vi "DropVI_SimpleClientPublisher.vi"() -> ()   [LabVIEW 2013, in "MQTT Client.lvlib"]
uses:
  MQTT Client.lvlib
  <vilib>/LabVIEW Open Source Project/MQTT Connection/MQTT_Connection/Connection/Connection.lvclass
  Client class/Client.lvclass/Client.ctl
  <vilib>/LabVIEW Open Source Project/MQTT Connection/MQTT_Base/Base Class/MQTT_Base.lvclass/MQTT_Base.ctl
  <vilib>/LabVIEW Open Source Project/MQTT Control Packets/Control Packets/PUBLISH/PUBLISH.lvclass
  Client class/Client.lvclass
  <vilib>/LabVIEW Open Source Project/MQTT Connection/MQTT_Base/Base Class/MQTT_Base.lvclass
panel:
  out "last error":errorcluster
  in  "Connection":bool
  out "Waveform Chart":dbl(graph)
  out "Published":bool
  in  "Stop Client":bool
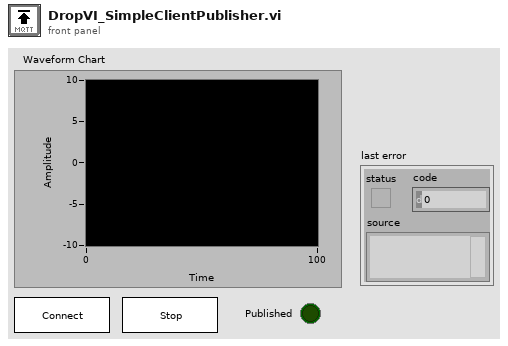
[diagram p1: front panel]
types:
  T1 = typedef "MQTT Client.lvlib/Client.lvclass/Public Events -- cluster.ctl" = cluster{"Connection Status":refnum<user-event>, "Connected":refnum<user-event>, "Application Message":refnum<user-event>}
  T2 = typedef "MQTT Base.lvlib/MQTT_Base.lvclass/Public Events -- cluster.ctl" = cluster{"Stop Event":refnum<user-event>, "Error Event":refnum<user-event>, "Inbound Message":refnum<user-event>}
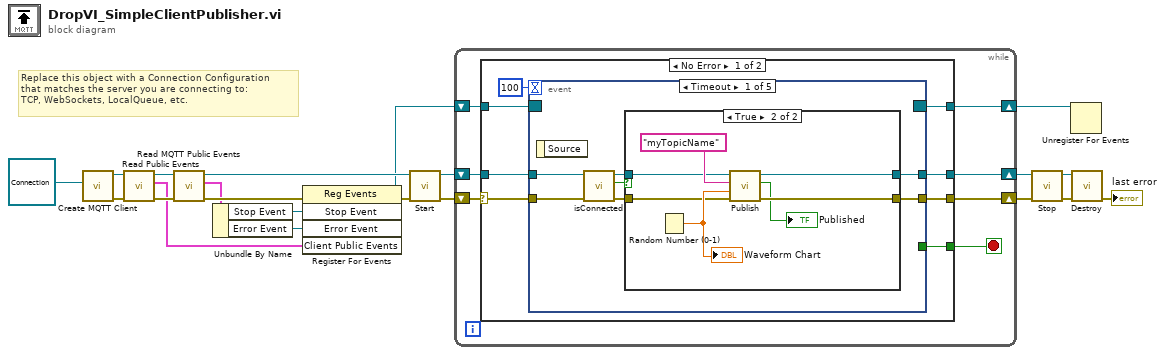
[diagram p0: block diagram]
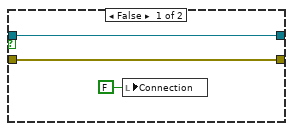
[diagram p2: hidden frame]
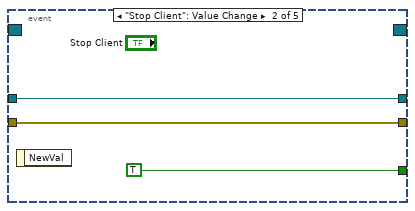
[diagram p3: hidden frame]
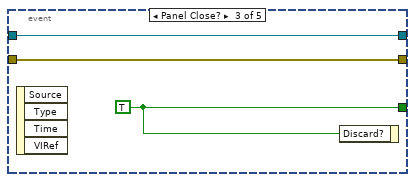
[diagram p4: hidden frame]
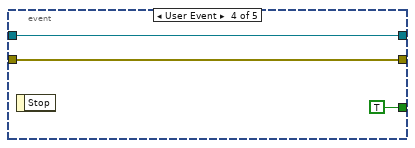
[diagram p5: hidden frame]
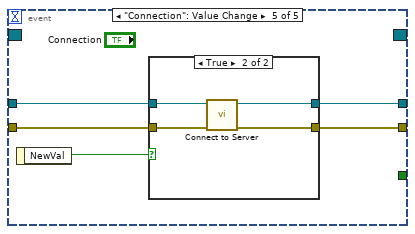
[diagram p6: hidden frame]
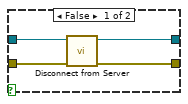
[diagram p7: hidden frame]
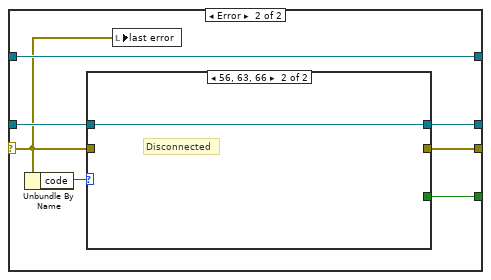
[diagram p8: hidden frame]
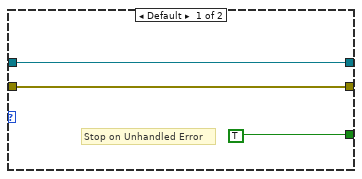
[diagram p9: hidden frame]
diagram:
  # "Replace this object with a Connection Configuration\nthat matches the server you are connecting to:\nTCP, WebSockets, LocalQueue, etc."
  n1 = call "Create MQTT Client.vi"("Connection Configuration"=refnum<class "Connection.lvclass"> refnum) -> ("error out"=w19:errorcluster, "Client out"=w21:refnum<class "Client.lvclass">)  [unwired: 9 in]
  n2 = call "Read Public Events.vi"("error in (no error)"=w19, "Client in"=w21) -> ("error out"=w18:errorcluster, "Client Public Events"=w16:T1, "Client out"=w20:refnum<class "Client.lvclass">)  [unwired: 7 in]
  n3 = call <vilib>:"Read MQTT Public Events.vi"("error in (no error)"=w18, "MQTT_Base in"=w20) -> ("error out"=w17:errorcluster, "MQTT Public Events"=w9:T2, "MQTT_Base out"=w14:refnum<class "Client.lvclass">)  [unwired: 7 in]
  n4 = Unbundle By Name(w9) -> ("Stop Event"=w11:refnum<user-event>, "Error Event"=w10:refnum<user-event>)
  n5 = register-events(error in=w17, w11, w10, w16) -> (reference out=w13:refnum<event-registration>, error out=w15:errorcluster)  [unwired: 1 in]
  n6 = call <vilib>:"Start.vi"("error in (no error)"=w15, "MQTT_Base in"=w14) -> ("error out"=w2:errorcluster, "MQTT_Base out"=w3:refnum<class "Client.lvclass">)  [unwired: 7 in, 1 out]
  n7 = while {
    shift-right: [w27] -> w12
    shift-left: w13 -> [w28]
    shift-right: [w24] -> w6
    shift-left: w3 -> [w25]
    shift-right: [w26] -> w4
    shift-left: w2 -> [w22]
    stop <- w23 stop-if-true
    n8 = case shown="No Error" w22 {
      selector: w22 -> [w29 w76]
      tunnel: w28 -> [w36 w82]
      tunnel: [w35 w82] -> w27
      tunnel: [w34 w78] -> w26
      tunnel: w25 -> [w32 w80]
      tunnel: [w31 w79] -> w24
      tunnel: [w30 w77] -> w23
      frame No Error {
        n9 = event shown="[0] Timeout" {
          selector: w36 -> [_ _ _ _ _]
          dyn-events: [_ _ _ _ _] -> w35
          timeout: 100 -> [_ _ _ _ _]
          tunnel: w29 -> [w39 w55 w57 w62 w63]
          tunnel: [w42 w55 w57 w62 w64] -> w34
          tunnel: [_ TRUE w59 TRUE _] -> w30
          tunnel: w32 -> [w41 w56 w58 w60 w67]
          tunnel: [w43 w56 w58 w60 w65] -> w31
          event Timeout {
            n10 = event-data() -> ()  [unwired: 1 in, 1 out]
            n11 = call "isConnected.vi"("error in (no error)"=w39, "Client in"=w41) -> ("error out"=w38:errorcluster, "connected"=w37:bool, "Client out"=w40:refnum<class "Client.lvclass">)  [unwired: 7 in]
            n12 = case shown="True" w37 {
              tunnel: [w46 w52] -> w43
              tunnel: [w45 w51] -> w42
              tunnel: w40 -> [w46 w48]
              tunnel: w38 -> [w45 w47]
              frame False {
                n13 = local write "Connection"(FALSE ("Connection")) -> ()
              }
              frame True {
                n14 = Random Number (0-1)() -> (number: 0 to 1=w49:dbl)
                "Waveform Chart" <- w49
                n15 = call "Publish.vi"("error in (no error)"=w47, "Payload"=w49, "Topic Name (empty: Payload name)"="myTopicName", "Client in"=w48) -> ("error out"=w51:errorcluster, "Published"=→"Published":bool, "Client out"=w52:refnum<class "Client.lvclass">)  [unwired: 5 in]
              }
            }
          }
          event "Stop Client": Value Change {
            n16 = event-data() -> ()  [unwired: 1 in, 1 out]
          }
          event Panel Close? {
            w59 = TRUE
            n17 = event-data() -> ()  [unwired: 1 in, 4 out]
            n18 = event-data("Discard?"=w59) -> ()  [unwired: 1 in, 1 out]
          }
          event User Event {
            n19 = event-data() -> ()  [unwired: 1 in, 1 out]
          }
          event "Connection": Value Change {
            n20 = event-data() -> ("NewVal"=w66:bool)  [unwired: 1 in]
            n21 = case shown="True" w66 {
              tunnel: w67 -> [w71 w75]
              tunnel: [w70 w72] -> w65
              tunnel: [w69 w73] -> w64
              tunnel: w63 -> [w68 w74]
              frame False {
                n22 = call "Disconnect from Server.vi"("error in (no error)"=w68, "Client in"=w71) -> ("error out"=w69:errorcluster, "Client out"=w70:refnum<class "Client.lvclass">)  [unwired: 7 in, 1 out]
              }
              frame True {
                n23 = call "Connect to Server.vi"("error in (no error)"=w74, "Client in"=w75) -> ("error out"=w73:errorcluster, "Client out"=w72:refnum<class "Client.lvclass">)  [unwired: 6 in, 2 out]
              }
            }
          }
        }
      }
      frame Error {
        n24 = Unbundle By Name(w76) -> ("code"=w81:i32)
        n25 = case shown="56, 63, 66" w81 {
          tunnel: w80 -> [w85 w86]
          tunnel: [w85 w86] -> w79
          tunnel: w76 -> [w84 _]
          tunnel: [w84 _] -> w78
          tunnel: [TRUE _] -> w77
          frame Default {
            # "Stop on Unhandled Error"
          }
          frame 56, 63, 66 {
            # "Disconnected"
          }
        }
        n26 = local write "last error"(w76) -> ()
      }
    }
  }
  n27 = call <vilib>:"Stop.vi"("error in (no error)"=w4, "MQTT_Base in"=w6) -> ("error out"=w5:errorcluster, "MQTT_Base out"=w7:refnum<class "Client.lvclass">)  [unwired: 7 in, 1 out]
  n28 = Unregister For Events(event registration refnum=w12) -> ()  [unwired: 1 in, 1 out]
  n29 = call <vilib>:"Destroy.vi"("error in (no error)"=w5, "MQTT_Base in"=w7) -> ("error out"=→"last error":errorcluster)  [unwired: 8 in, 1 out]
